vi "FinalLabview.vi"() -> ()   [LabVIEW 2020]
uses:
  <vilib>/httpClient/POSTBuffer.vi
  <vilib>/ptbypt/NI_PtbyPt.lvlib
  <vilib>/httpClient/LabVIEWHTTPClient.lvlib
  <vilib>/smtpClient/LabVIEWSMTPClient.lvlib
panel:
  out "Boolean":bool
  out "resulting string":string
  out "JSON string":string
  in  "Cluster":cluster{"temperature":dbl, "humidity":dbl}
  out "Pump Duration":dbl
  out "Pot ID":dbl
  in  "Max Pump Time":dbl
  in  "K Value":dbl
  in  "Target Moisture":dbl
  in  "Hhigh":dbl
  in  "Hlow":dbl
  in  "Vwet":dbl
  in  "Vdry":dbl
  out "Pot Website Status":string
  out "Soil Condition":string
  out "Selected Soil Voltage":dbl
  out "Moisture %":dbl(knob) scale=0.0..100.0
  out "Environment Website Status":string
  out "Humidity (V)":dbl format="%#_2g"
  out "Temperature (V)":dbl format="%#_2g"
  out "Humidity %":dbl(knob) scale=0.0..100.0
  out "Temperature °C":dbl(slide) scale=0.0..100.0
  out "Pot Number From Robot":dbl
  out "Pot Bit 1":bool
  out "Pot Bit 0":bool
  out "Robot Stop Detected":bool
  out "Data Uploaded Already":bool
  in  "stop":bool
  # "SMART GARDEN ROBOT"
  # "Live Environment"
  # "Selected Pot Data"
  # "Robot Input"
  # "System Status"
  # "Calibration Settings"
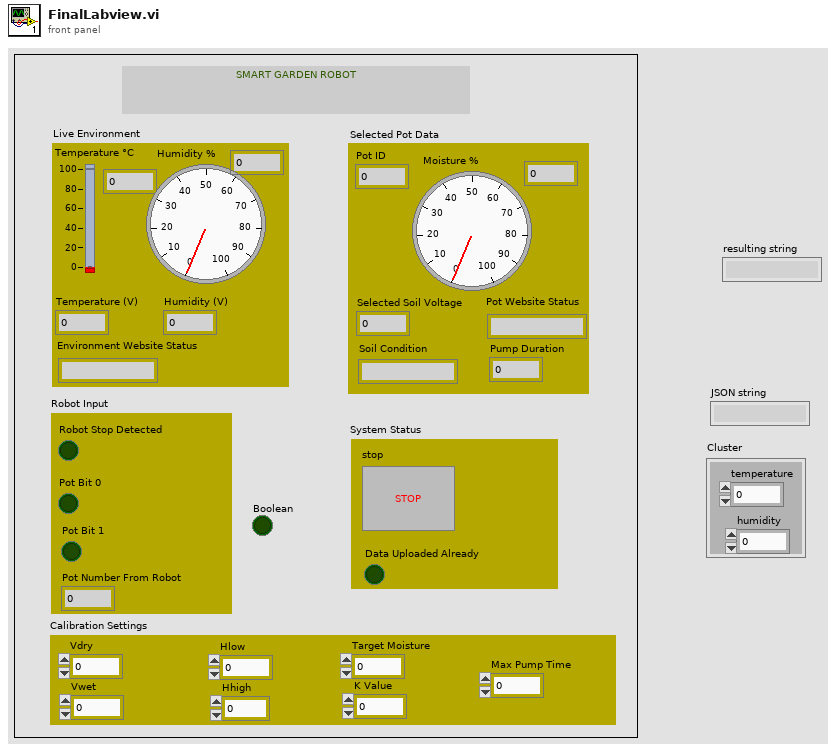
[diagram p1: front panel]
types:
  T1 = typedef "LabVIEWHTTPClient.lvlib/ClientHandle.ctl" = refnum<k1>
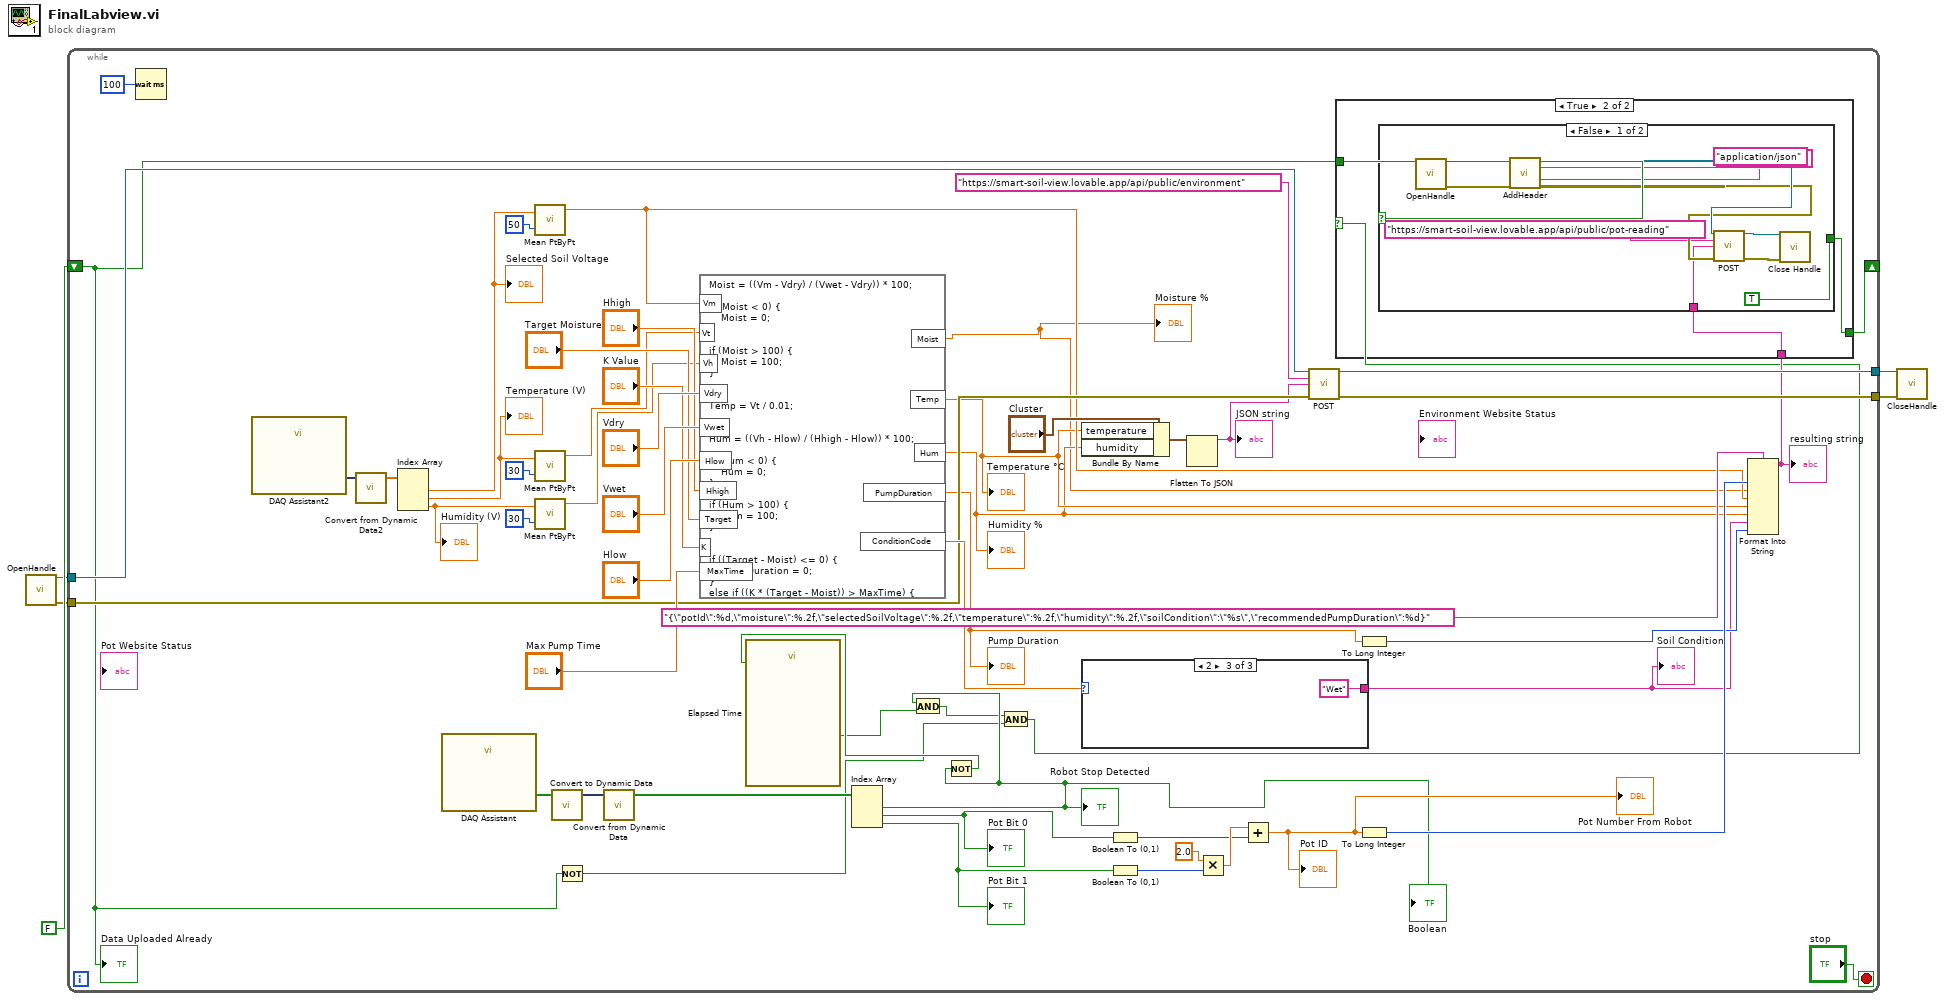
[diagram p0: block diagram]
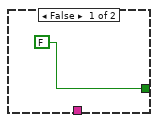
[diagram p2: hidden frame]
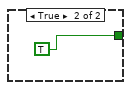
[diagram p3: hidden frame]
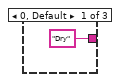
[diagram p4: hidden frame]
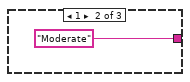
[diagram p5: hidden frame]
diagram:
  n1 = call <vilib>:"OpenHandle.vi"() -> ("client handle out"=w4:T1, "error out"=w3:errorcluster)  [unwired: 14 in]
  n2 = while {
    shift-right: [w15] -> _
    shift-left: FALSE -> [w11]
    tunnel: w4 -> [w32]
    tunnel: w3 -> [w31]
    tunnel: [w26] -> w2
    tunnel: [w25] -> w1
    stop <- "stop" stop-if-true
    n3 = Wait (ms)(milliseconds to wait=u32 100) -> ()  [unwired: 1 out]
    n4 = call "DAQ Assistant2"() -> ("data"=w50:dynamicdata)  [unwired: 17 in, 2 out]
    n5 = call "Convert from Dynamic Data2"("Dynamic Data Type"=w50) -> ("Array"=w49:dbl[])  [unwired: 3 in]
    n6 = Index Array(array=w49) -> (element #1=w38:dbl, element #2=w40:dbl, element #3=w37:dbl)  [unwired: 3 in]
    "Selected Soil Voltage" <- w38
    "Temperature (V)" <- w40
    "Humidity (V)" <- w37
    n7 = call "DAQ Assistant"() -> ("data"=w59:bool[])  [unwired: 17 in, 2 out]
    n8 = call <vilib>:"Mean PtByPt.vi"("x"=w38, "sample length"=50) -> ("mean"=w19:dbl)  [unwired: 2 in, 1 out]
    n9 = call <vilib>:"Mean PtByPt.vi"("x"=w40, "sample length"=30) -> ("mean"=w39:dbl)  [unwired: 2 in, 1 out]
    n10 = call <vilib>:"Mean PtByPt.vi"("x"=w37, "sample length"=30) -> ("mean"=w36:dbl)  [unwired: 2 in, 1 out]
    n11 = call "Convert to Dynamic Data"("Array"=w59) -> ("Dynamic Data Type"=w58:dynamicdata)  [unwired: 3 in]
    n12 = Not(x=w11) -> (.not. x?=w7:bool)
    n13 = call "Convert from Dynamic Data"("Dynamic Data Type"=w58) -> ("Array"=w57:bool[])  [unwired: 3 in]
    n14 = formula code="Moist = ((Vm - Vdry) / (Vwet - Vdry)) * 100;\n\nif (Moist < 0) {\n    Moist = 0;\n}\n\nif (Moist > 100) {\n    Moist = 100;\n}\n\n\nTemp = Vt / 0.01;\n\n\nHum = ((Vh - Hlow) / (Hhigh - Hlow)) * 100;\n\nif (Hum < 0) {\n    Hum = 0;\n}\n\nif (Hum > 100) {\n    Hum = 100;\n}\n\n\nif ((Target - Moist) <= 0) {\n    PumpDuration = 0;\n}\nelse if ((K * (Target - Moist)) > MaxTime) {\n    \n    if (MaxTime <= 0) {\n        PumpDuration = 0;\n    }\n    else if (MaxTime <= 2) {\n        PumpDuration = 2;\n    }\n    else if (MaxTime <= 4) {\n        PumpDuration = 4;\n    }\n    else {\n        PumpDuration = 8;\n    }\n}\nelse if ((K * (Target - Moist)) <= 2) {\n    PumpDuration = 2;\n}\nelse if ((K * (Target - Moist)) <= 4) {\n    PumpDuration = 4;\n}\nelse {\n    PumpDuration = 8;\n}\n\n\nif (Moist < 40) {\n    ConditionCode = 0;\n}\nelse if (Moist < 60) {\n    ConditionCode = 1;\n}\nelse {\n    ConditionCode = 2;\n}"("Vm"=w19, "Vt"=w39, "Vh"=w36, "Vdry"="Vdry", "Vwet"="Vwet", "Hlow"="Hlow", "Hhigh"="Hhigh", "Target"="Target Moisture", "K"="K Value", "MaxTime"="Max Pump Time") -> ("Moist"=w13:dbl, "Temp"=w18:dbl, "Hum"=w17:dbl, "PumpDuration"=w22:dbl, "ConditionCode"=w41:dbl)
    "Moisture %" <- w13
    "Humidity %" <- w17
    "Temperature °C" <- w18
    "Pump Duration" <- w22
    n15 = Index Array(array=w57) -> (element #1=w9:bool, element #2=w56:bool, element #3=w55:bool)  [unwired: 3 in]
    "Robot Stop Detected" <- w9
    "Pot Bit 0" <- w56
    "Pot Bit 1" <- w55
    "Boolean" <- w9
    n16 = Not(x=w9) -> (.not. x?=w12:bool)
    n17 = call "Elapsed Time"("Reset"=w12) -> ("Time has Elapsed"=w10:bool)  [unwired: 11 in, 7 out]
    n18 = And(x=w9, y=w10) -> (x .and. y?=w8:bool)
    n19 = And(x=w8, y=w7) -> (x .and. y?=w6:bool)
    n20 = Bundle By Name(cluster="Cluster", "temperature"=w18, "humidity"=w17) -> (w29:cluster{"temperature":dbl, "humidity":dbl})
    n21 = case shown="2" w41 {
      tunnel: ["Dry" "Moderate" "Wet"] -> w16
      frame 0, Default {
      }
      frame 1 {
      }
      frame 2 {
      }
    }
    "Soil Condition" <- w16
    n22 = Boolean To (0,1)(Boolean=w56) -> (0, 1=w51:i16)
    n23 = Boolean To (0,1)(Boolean=w55) -> (0, 1=w52:i16)
    n24 = Flatten To JSON(anything=w29) -> (JSON string=w28:string)  [unwired: 2 in, 1 out]
    "JSON string" <- w28
    n25 = Multiply(x=2.0, y=w52) -> (x*y=w54:dbl)
    n26 = Add(x=w54, y=w51) -> (x+y=w23:dbl)
    "Pot ID" <- w23
    "Pot Number From Robot" <- w23
    n27 = call-poly <vilib>:"POST.vi"("client handle"=w32, "url"="https://smart-soil-view.lovable.app/api/public/environment", "buffer"=w28, "error in (no error)"=w31) -> ("client handle out"=w26:T1, "error out"=w25:errorcluster)  [unwired: 8 in, 2 out]
    n28 = To Long Integer(number=w22) -> (32bit integer=w20:i32)
    n29 = To Long Integer(number=w23) -> (32bit integer=w21:i32)
    n30 = Format Into String(format string="{\"potId\":%d,\"moisture\":%.2f,\"selectedSoilVoltage\":%.2f,\"temperature\":%.2f,\"humidity\":%.2f,\"soilCondition\":\"%s\",\"recommendedPumpDuration\":%d}", w21, w13, w19, w18, w17, w16, w20) -> (resulting string=w14:string)  [unwired: 2 in, 1 out]
    "resulting string" <- w14
    n31 = case shown="True" w6 {
      tunnel: [FALSE w64] -> w15
      tunnel: w11 -> [_ w65]
      tunnel: w14 -> [_ w63]
      frame False {
      }
      frame True {
        n32 = case shown="False" w65 {
          tunnel: [TRUE TRUE] -> w64
          tunnel: w63 -> [w66 _]
          frame False {
            n33 = call <vilib>:"OpenHandle.vi"() -> ("client handle out"=w75:T1, "error out"=w72:errorcluster)  [unwired: 14 in]
            n34 = call <vilib>:"AddHeader.vi"("client handle"=w75, "header"="Content-Type", "value"="application/json", "error in (no error)"=w72) -> ("client handle out"=w74:T1, "error out"=w71:errorcluster)  [unwired: 10 in]
            n35 = call-poly <vilib>:"POST.vi"("client handle"=w74, "url"="https://smart-soil-view.lovable.app/api/public/pot-reading", "buffer"=w66, "error in (no error)"=w71) -> ("client handle out"=w73:T1, "error out"=w70:errorcluster)  [unwired: 8 in, 2 out]
            n36 = call <vilib>:"Close Handle.vi"("handle in"=w73, "error in (no error)"=w70) -> ()  [unwired: 12 in, 2 out]
          }
          frame True {
          }
        }
      }
    }
    "Data Uploaded Already" <- w11
  }
  n37 = call <vilib>:"CloseHandle.vi"("client handle"=w2, "error in (no error)"=w1) -> ()  [unwired: 13 in, 1 out]
